vi "Pressure_statistic with temperature(multiple regime)+SR810.vi"() -> ()   [LabVIEW 2014]
uses:
  <vilib>/Utility/error.llb/DialogType.ctl
  Instance          11 26Saved   Pressure_statistic .vi
  Instance           2 26Saved   Pressure_statistic .vi
  Instance           9 26Saved   Pressure_statistic .vi
  Instance           8 26Saved   Pressure_statistic .vi
  <instrlib>/Stanford Research 830/Public/Data/Read (Multiple Points).vi
  Instance           7 26Saved   Pressure_statistic .vi
  Instance           5 26Saved   Pressure_statistic .vi
  <vilib>/Utility/file.llb/Write To Spreadsheet File (DBL).vi
  Instance           4 26Saved   Pressure_statistic .vi
  <instrlib>/Fluke 884X Series/Public/Data/Read (Multiple Points).vi
  Instance          16 26Saved   Pressure_statistic .vi
  <instrlib>/Fluke 884X Series/Fluke 884X Series.lvlib
  Downloads/stanford_research_830 (1)/Stanford Research 830/Stanford Research 830.lvlib
panel:
  in  "Number of Points (100)":u32=100
  in  "Sample Rate (10: 64 Hz)":u16(ring)=10 items=["62.5 mHz", "125 mHz", "250 mHz", "500 mHz", "1 Hz", "2 Hz", "4 Hz", "8Hz", "16 Hz", "32 Hz", "64 Hz", "128 Hz", "256 Hz", "512 Hz", "Trigger "]
  in  "Channel 1 Display (0: X)":u16(ring) items=["X", "R", "X Noise", "Aux In 1", "Aux In 2"]
  in  "Internal Reference Frequency (1000 Hz)":dbl=1000.0
  in  "Sine Output Amplitude (1 V)":dbl=1.0
  in  "Reference Source (1: Internal)":u16(ring)=1 items=["External", "Internal"]
  in  "Input Coupling (0: AC)":u16(ring) items=["AC", "DC"]
  in  "Input Connection (0: Single-Ended Voltage)":u16(ring) items=["Single-Ended Voltage", "Differential Voltage", "1 MOhm Current Gain", "100 MOhm Current Gain"]
  in  "VISA resource for sr810":refnum<visa-resource-name>
  in  "mkv per degree(thermocouple type)":dbl
  out "T,C":dbl
  out "T,K":dbl
  in  "Tkomn, C":dbl
  in  "Timeout":i32=10000
  in  "Sample Count (10)":i32=10
  in  "Manual Range (1.0)":dbl=1.0
  in  "Auto Range (T:Enable)":bool=TRUE
  in  "Function (0: DC Voltage)":u16(ring) items=["DC Voltage", "AC Voltage", "2 - Wire Resistance", "4 - Wire Resistance", "DC Current", "AC Current", "Frequency", "Period", "Continuity", "Diode Checking", "Temperature", "Capacitance"]
  in  "Manual Resolution (5.5 Digits)":dbl(ring)=5.5 items=["4.5"=4.5, "5.5"=5.5, "6.5"=6.5]
  out "Temperature":dbl
  out "Temperature from Fluke884X":dbl[](graph)
  in  "VISA resource for fluke":refnum<visa-resource-name>
  in  "Serial Configuration":T1={"Baud Rate"=9600, "Parity"=0, "Data Bits"=8, "Stop Bits"=10, "Flow Control"=0} {"Flow Control" items=["None", "XON/XOFF", "RTS/CTS", "XON/XOFF & RTS/CTS", "DTR/DSR", "XON/XOFF & DTR/DSR"]; "Stop Bits" items=["1.0"=10, "1.5"=15, "2.0"=20]; "Data Bits" items=["7"=7, "8"=8]; "Parity" items=["None", "Odd", "Even", "Mark", "Space"]; "Baud Rate" items=["300"=300, "600"=600, "1200"=1200, "2400"=2400, "4800"=4800, "9600"=9600, "19200"=19200]}
  in  "Filter 2":bool
  in  "Case Constant\n(See Context Help)":bool=TRUE
  in  "Write":bool
  out "P, V":dbl[](array[numeric])
  out "Waveform Graph 2":dbl[](graph)
  out "Waveform Graph":dynamicdata(graph)
  in  "Fourier transform":bool
  out "Pressure Frequency":dbl
  out "Pressure Amplitude":dbl
  in  "Filter":bool
  in  "Fourier transform":bool
  in  "Write to file":bool
  in  "stop":bool
  # "Responce"
  # "Pressure"
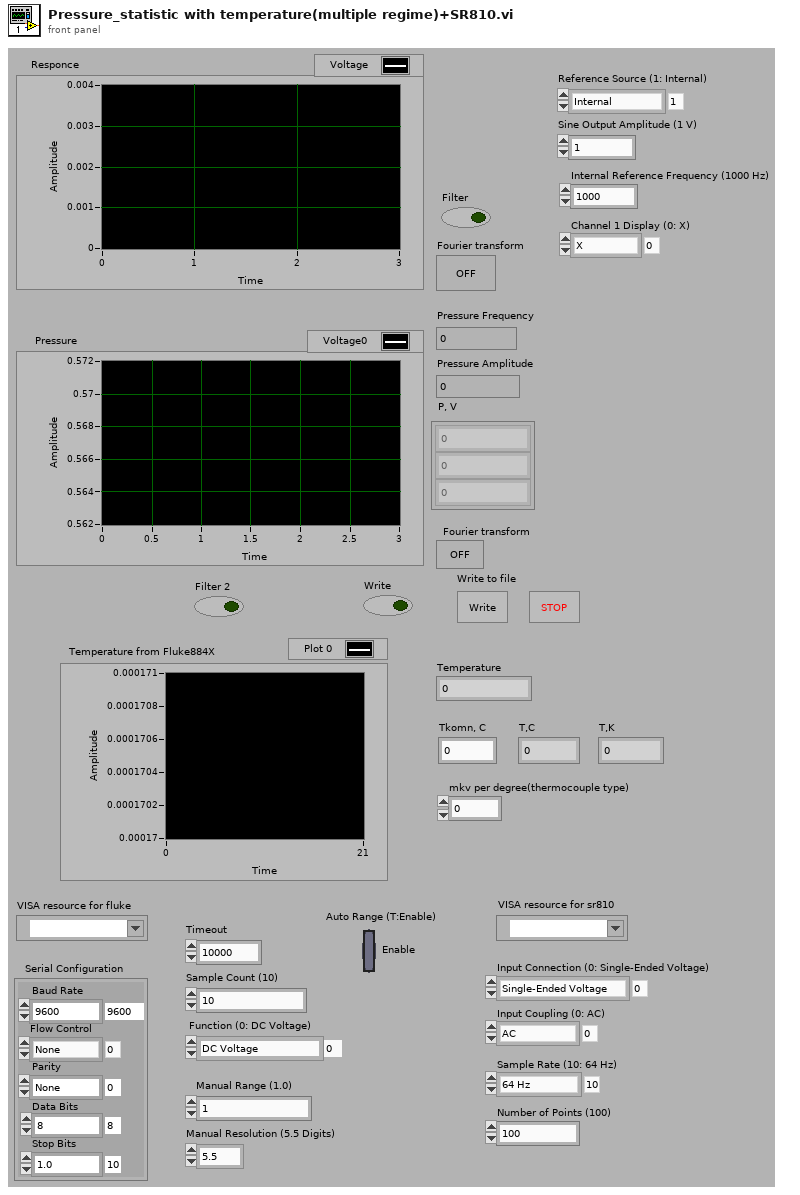
[diagram p1: front panel]
types:
  T1 = cluster{"Baud Rate":u32, "Parity":u16, "Data Bits":u16, "Stop Bits":u16, "Flow Control":u16}
  T2 = typedef "DialogType.ctl" = u16
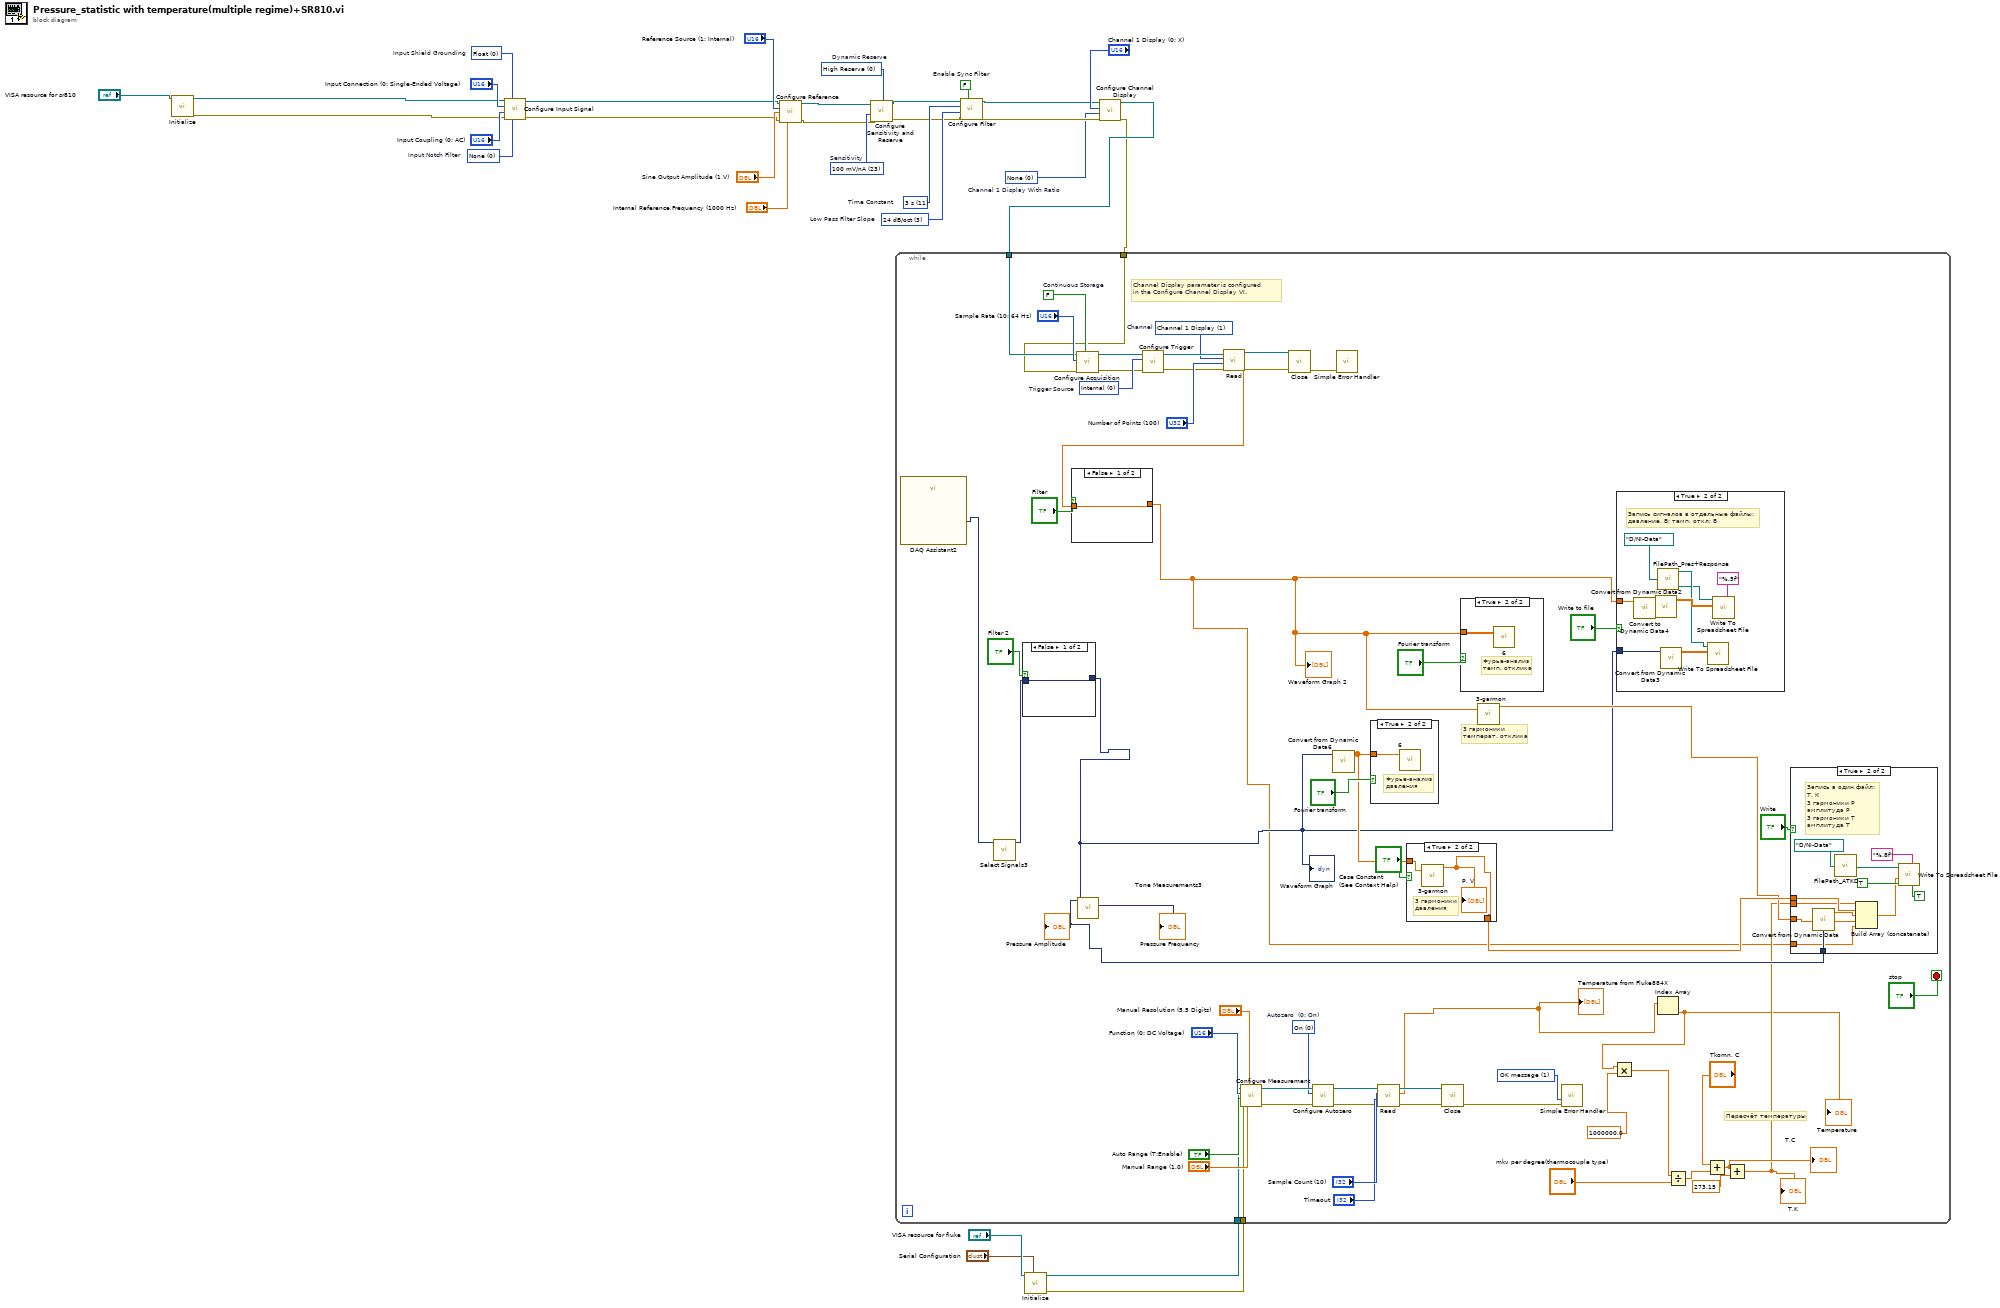
[diagram p0: block diagram]
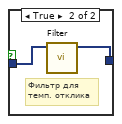
[diagram p2: hidden frame]
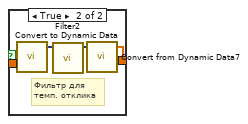
[diagram p6: hidden frame]
diagram:
  w3 = u16 0 items=["None", "Aux In 1", "Aux In 2"]  # Channel 1 Display With Ratio
  w10 = FALSE  # Enable Sync Filter
  w9 = u16 3 items=["6 dB/oct", "12 dB/oct", "18 db/oct", "24 dB/oct"]  # Low Pass Filter Slope
  w11 = u16 11 items=["10 us", "30 us", "100 us", "300 us", "1 ms", "3 ms", "10 ms", "30 ms", "100 ms", "300 ms", "1 s", "3 s", "10 s", "30 s", "100 s", "300 s", "1 ks", "3 ks", "10 ks", "30 ks"]  # Time Constant
  w15 = i16 23 items=["Auto Gain"=-1, "2 nV/fA"=0, "5 nV/fA"=1, "10 nV/fA"=2, "20 nV/fA"=3, "50 nV/fA"=4, "100 nV/fA"=5, "200 nV/fA"=6, "500 nV/fA"=7, "1 uV/pA"=8, "2 uV/pA"=9, "5 uV/pA"=10, "10 uV/pA"=11, "20 uV/pA"=12, "50 uV/pA"=13, "100 uV/pA"=14, "200 uV/pA"=15, "500 uV/pA"=16, "1 mV/nA"=17, "2 mV/nA"=18, "5 mV/nA"=19, "10 mV/nA"=20, "20 mV/nA"=21, "50 mV/nA"=22, "100 mV/nA"=23, "200 mV/nA"=24, "500 mV/mA"=25, "1 V/uA"=26]  # Sensitivity
  w14 = i16 0 items=["Auto Reserve"=-1, "High Reserve"=0, "Normal"=1, "Low Noise"=2]  # Dynamic Reserve
  w23 = u16 0 items=["None", "Line Notch", "2x Line Notch", "Both Notch Filters"]  # Input Notch Filter
  w26 = u16 0 items=["Float", "Ground"]  # Input Shield Grounding
  n1 = call <instrlib>:"Initialize.vi"("VISA resource name"="VISA resource for sr810") -> ("error out"=w21:errorcluster, "VISA resource name out"=w22:refnum<visa-resource-name>)  [unwired: 9 in]
  n2 = call "Configure Input Signal.vi"("Input Notch Filter (0: None)"=w23, "Input Shield Grounding (0: Float)"=w26, "error in (no error)"=w21, "Input Coupling (0: AC)"="Input Coupling (0: AC)", "Input Connection (0: Single-Ended Voltage)"="Input Connection (0: Single-Ended Voltage)", "VISA resource name"=w22) -> ("error out"=w16:errorcluster, "VISA resource name out"=w17:refnum<visa-resource-name>)  [unwired: 4 in]
  n3 = call "Configure Reference.vi"("VISA resource name"=w17, "Reference Source (1: Internal)"="Reference Source (1: Internal)", "Sine Output Amplitude (1 V)"="Sine Output Amplitude (1 V)", "error in (no error)"=w16, "Internal Reference Frequency (1000 Hz)"="Internal Reference Frequency (1000 Hz)") -> ("VISA resource name out"=w13:refnum<visa-resource-name>, "error out"=w12:errorcluster)  [unwired: 9 in]
  n4 = call "Configure Sensitivity and Reserve.vi"("error in (no error)"=w12, "Sensitivity (-1: Auto gain)"=w15, "Dynamic Reserve (-1: Auto Reserve)"=w14, "VISA resource name"=w13) -> ("error out"=w7:errorcluster, "VISA resource name out"=w8:refnum<visa-resource-name>)  [unwired: 6 in]
  n5 = call "Configure Filter.vi"("Enable Sync Filter (F: Disable)"=w10, "error in (no error)"=w7, "Low Pass Filter Slope (1: 12dB/oct)"=w9, "Time Constant (8: 100ms)"=w11, "VISA resource name"=w8) -> ("error out"=w5:errorcluster, "VISA resource name out"=w4:refnum<visa-resource-name>)  [unwired: 5 in]
  n6 = call <instrlib>:"Initialize.vi"("Serial Configuration"="Serial Configuration", "VISA resource name"="VISA resource for fluke") -> ("error out"=w30:errorcluster, "VISA resource name out"=w31:refnum<visa-resource-name>)  [unwired: 8 in]
  n7 = call "Configure Channel Display.vi"("error in (no error)"=w5, "Channel 1 Display With Ratio (0: None)"=w3, "Channel 1 Display (0: X)"="Channel 1 Display (0: X)", "VISA resource name"=w4) -> ("error out"=w1:errorcluster, "VISA resource name out"=w2:refnum<visa-resource-name>)  [unwired: 6 in]
  n8 = while {
    tunnel: w31 -> [w60]
    tunnel: w30 -> [w59]
    tunnel: w2 -> [w35]
    tunnel: w1 -> [w34]
    stop <- "stop" stop-if-true
    w38 = u16 1 items=["Channel 1 Display"=1, "Channel 2 Display"=2]  # Channel
    w46 = u16 0 items=["Internal", "External"]  # Trigger Source
    w37 = FALSE  # Continuous Storage
    w61 = u16 0 items=["On", "Off", "Once"]  # Autozero  (0: On)
    w75 = T2 1 items=["no dialog", "OK message", "continue or stop message", "OK message + warnings", "continue/stop + warnings"] ("type of dialog (OK msg:1)")
    # "Channel Display parameter is configured\nin the Configure Channel Display VI."
    # "Пересчёт температуры"
    # "3 гармоники\nтемперат. отклика"
    n9 = call "DAQ Assistant2"() -> ("data"=w85:dynamicdata)  [unwired: 2 in, 9 out]
    n10 = call "Select Signals3"("Signals"=w85) -> ("Signal Out"=w78:dynamicdata)  [unwired: 1 in, 9 out]
    n11 = case shown="False" "Filter 2" {
      tunnel: w78 -> [w91 w93]
      tunnel: [w91 w92] -> w76
      frame False {
      }
      frame True {
        # "Фильтр для\nтемп. отклика"
        n12 = call "Filter"("Signal"=w93) -> ("Filtered Signal"=w92:dynamicdata)  [unwired: 2 in, 8 out]
      }
    }
    "Waveform Graph" <- w76
    n13 = call "Configure Acquisition.vi"("Continuous Storage (T: Enable)"=w37, "error in (no error)"=w34, "Sample Rate (0: 62.5 mHz)"="Sample Rate (10: 64 Hz)", "VISA resource name"=w35) -> ("error out"=w44:errorcluster, "VISA resource name out"=w45:refnum<visa-resource-name>)  [unwired: 6 in]
    n14 = call "Tone Measurements3"("Signals"=w76) -> ("Frequency"=→"Pressure Frequency":dynamicdata, "Amplitude"=w79:dynamicdata)  [unwired: 1 in, 8 out]
    "Pressure Amplitude" <- w79
    n15 = call "Configure Trigger.vi"("error in (no error)"=w44, "Trigger Source (0: Internal)"=w46, "VISA resource name"=w45) -> ("error out"=w41:errorcluster, "VISA resource name out"=w42:refnum<visa-resource-name>)  [unwired: 7 in]
    n16 = call-poly <instrlib>:"Read.vi"("error in (no error)"=w41, "Number of Points (100)"="Number of Points (100)", "Channel (1: Channel 1 Display)"=w38, "VISA resource name"=w42) -> ("error out"=w39:errorcluster, "Measurements"=w33:sgl[], "VISA resource name out"=w40:refnum<visa-resource-name>)  [unwired: 5 in]
    n17 = case shown="False" "Filter" {
      tunnel: w33 -> [w109 w113]
      tunnel: [w109 w111] -> w32
      frame False {
      }
      frame True {
        # "Фильтр для\nтемп. отклика"
        n18 = call "Convert to Dynamic Data"("Array"=w113) -> ("Dynamic Data Type"=w110:dynamicdata)  [unwired: 3 in]
        n19 = call "Filter2"("Signal"=w110) -> ("Filtered Signal"=w112:dynamicdata)  [unwired: 2 in, 8 out]
        n20 = call "Convert from Dynamic Data7"("Dynamic Data Type"=w112) -> ("Array"=w111:dbl[])  [unwired: 3 in]
      }
    }
    "Waveform Graph 2" <- w32
    n21 = call <instrlib>:"Configure Measurement.vi"("Manual Range (1.0)"="Manual Range (1.0)", "Manual Resolution (5.5 Digits)"="Manual Resolution (5.5 Digits)", "error in (no error)"=w59, "Auto Range (T:Enable)"="Auto Range (T:Enable)", "Function (0: DC Voltage)"="Function (0: DC Voltage)", "VISA resource name"=w60) -> ("error out"=w65:errorcluster, "VISA resource name out"=w64:refnum<visa-resource-name>)  [unwired: 4 in]
    n22 = call <instrlib>:"Close.vi"("error in (no error)"=w39, "VISA resource name"=w40) -> ("error out"=w47:errorcluster)  [unwired: 9 in]
    n23 = call <instrlib>:"Configure Autozero.vi"("error in (no error)"=w65, "Autozero  (0: On)"=w61, "VISA resource name"=w64) -> ("error out"=w62:errorcluster, "VISA resource name out"=w63:refnum<visa-resource-name>)  [unwired: 7 in]
    n24 = call "Convert from Dynamic Data6"("Dynamic Data Type"=w76) -> ("Array"=w82:dbl[])  [unwired: 3 out]
    n25 = call <vilib>:"Simple Error Handler.vi"("error in (no error)"=w47) -> ()  [unwired: 4 in, 5 out]
    n26 = case shown="True" "Fourier transform" {
      tunnel: w82 -> [_ w108]
      frame False {
      }
      frame True {
        # "Фурье-анализ\nдавления"
        n27 = call "6.vi"("X"=w108) -> ()  [unwired: 7 out]
      }
    }
    n28 = call-poly <instrlib>:"Read.vi"("error in (no error)"=w62, "Timeout (10000 ms)"="Timeout", "Sample Count (1)"="Sample Count (10)", "VISA resource name"=w63) -> ("error out"=w72:errorcluster, "Measurements"=w54:dbl[], "VISA resource name out"=w73:refnum<visa-resource-name>)  [unwired: 5 in]
    "Temperature from Fluke884X" <- w54
    n29 = case shown="True" "Case Constant\n(See Context Help)" {
      tunnel: w82 -> [_ w107]
      tunnel: [_ w106] -> w81
      frame False {
      }
      frame True {
        # "3 гармоники\nдавления"
        n30 = call "3-garmon.vi"("X"=w107) -> ("A"=w106:dbl[])  [unwired: 6 out]
        "P, V" <- w106
      }
    }
    n31 = call <instrlib>:"Close.vi"("error in (no error)"=w72, "VISA resource name"=w73) -> ("error out"=w74:errorcluster)  [unwired: 9 in]
    n32 = case shown="True" "Fourier transform" {
      tunnel: w32 -> [_ w114]
      frame False {
      }
      frame True {
        # "Фурье-анализ\nтемп. отклика"
        n33 = call "6.vi"("X"=w114) -> ()  [unwired: 7 out]
      }
    }
    n34 = call "3-garmon.vi"("X"=w32) -> ("A"=w80:dbl[])  [unwired: 6 out]
    n35 = call <vilib>:"Simple Error Handler.vi"("type of dialog (OK msg:1)"=w75, "error in (no error)"=w74) -> ()  [unwired: 3 in, 5 out]
    n36 = case shown="True" "Write to file" {
      tunnel: w32 -> [_ w123]
      tunnel: w76 -> [_ w120]
      frame False {
      }
      frame True {
        # "Запись сигналов в отдельные файлы:\nдавление, В; темп. откл; В"
        n37 = call "Convert to Dynamic Data4"("Array"=w123) -> ("Dynamic Data Type"=w115:dynamicdata)  [unwired: 3 in]
        n38 = call "Convert from Dynamic Data2"("Dynamic Data Type"=w115) -> ("Array"=w122:dbl[][])  [unwired: 3 out]
        n39 = call "FilePath_Pres+Response.vi"("base folder path"=path "D:/NI-Data") -> ("Pressure"=w118:path, "Response"=w117:path)  [unwired: 1 out]
        n40 = call "Convert from Dynamic Data3"("Dynamic Data Type"=w120) -> ("Array"=w121:dbl[][])  [unwired: 3 out]
        n41 = call-poly <vilib>:"Write To Spreadsheet File.vi"("2D data"=w121, "file path (dialog if empty)"=w118) -> ()  [unwired: 4 in, 3 out]
        n42 = call-poly <vilib>:"Write To Spreadsheet File.vi"("format (%.3f)"="%.5f", "2D data"=w122, "file path (dialog if empty)"=w117) -> ()  [unwired: 3 in, 3 out]
      }
    }
    n43 = Index Array(array=w54) -> (element=w51:dbl)  [unwired: 1 in]
    "Temperature" <- w51
    n44 = Multiply(x=w51, y=1000000.0) -> (x*y=w49:dbl)
    n45 = Divide(x=w49, y="mkv per degree(thermocouple type)") -> (x/y=w57:dbl)
    n46 = Add(x="Tkomn, C", y=w57) -> (x+y=w55:dbl)
    "T,C" <- w55
    n47 = Add(x=w55, y=273.15) -> (x+y=w52:dbl)
    "T,K" <- w52
    n48 = case shown="True" "Write" {
      tunnel: w81 -> [_ w105]
      tunnel: w80 -> [_ w99]
      tunnel: w79 -> [_ w98]
      tunnel: w32 -> [_ w94]
      tunnel: w52 -> [_ w95]
      frame False {
      }
      frame True {
        # "Запись в один файл:\nТ, К\n3 гармоники P\nамплитуда P\n3 гармоники Т\nамплитуда Т"
        n49 = call "Convert from Dynamic Data"("Dynamic Data Type"=w98) -> ("Array"=w97:dbl[])  [unwired: 3 out]
        n50 = call "FilePath_ATKD.vi"("base folder path"=path "D:/NI-Data") -> ("ATKD"=w104:path)  [unwired: 3 out]
        n51 = Build Array (concatenate)(w95, w105, w97, w99, w94) -> (w96:dbl[])
        n52 = call-poly <vilib>:"Write To Spreadsheet File.vi"("transpose? (no:F)"=TRUE, "format (%.3f)"="%.8f", "append to file? (new file:F)"=TRUE, "1D data"=w96, "file path (dialog if empty)"=w104) -> ()  [unwired: 1 in, 3 out]
      }
    }
  }
